vi "Set pin status.vi"(7 "Value":bool, 8 "error in (no error)":errorcluster, 9 "Pin":dbl, 10 "Port":dbl, 11 "Simulado in":refnum<class "Simulado.lvclass">) -> (0 "error out":errorcluster, 3 "Simulado out":refnum<class "Simulado.lvclass">)   [LabVIEW 2020, in "Simulado.lvclass"]
uses:
  Simulado.lvclass
  Simulado.lvclass/Simulado.ctl
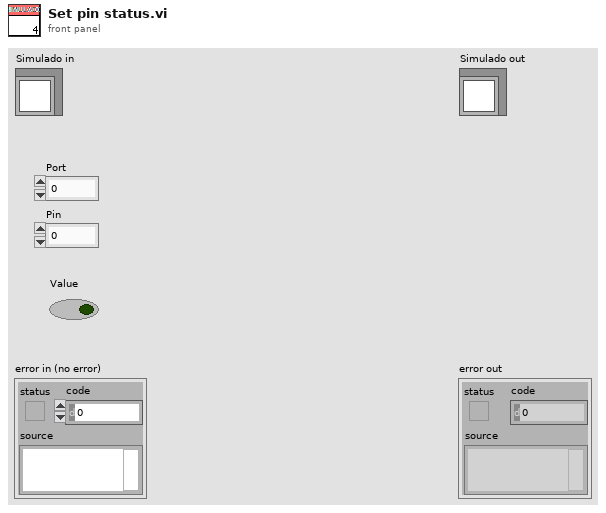
[diagram p1: front panel]
types:
  T1 = enum16{"reset parameters", "Get parameters", "Set parameter"}
  T2 = typedef "Serial Device.lvclass/serial device brand.ctl" = string
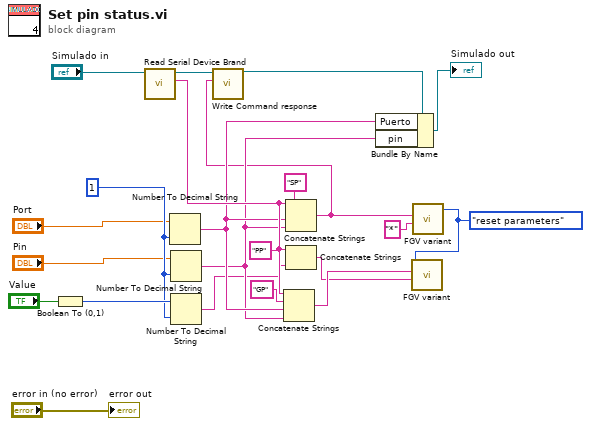
[diagram p0: block diagram]
diagram:
  w6 = T1."reset parameters" ("Functions")
  w15 = 1
  n1 = Boolean To (0,1)(Boolean="Value") -> (0, 1=w17:i16)
  n2 = call-dynamic "Read Serial Device Brand.vi"("Serial Device in"="Simulado in") -> ("Serial Device Brand"=w12:T2, "Serial Device out"=w21:refnum<class "Simulado.lvclass">)  [unwired: 8 in, 1 out]
  n3 = Number To Decimal String(number="Port", width (-)=w15) -> (decimal integer string=w8:string)
  n4 = Number To Decimal String(number="Pin", width (-)=w15) -> (decimal integer string=w7:string)
  n5 = Number To Decimal String(number=w17, width (-)=w15) -> (decimal integer string=w5:string)
  n6 = Concatenate Strings(w12, "GP" ("string"), w8, w7) -> (w3:string)
  n7 = Concatenate Strings(w12, "SP" ("string"), w8, w7) -> (w1:string)
  n8 = call-dynamic "Write Command response.vi"("Command response"=w1, "Simulado in"=w21) -> ("Simulado out"=w20:refnum<class "Simulado.lvclass">)  [unwired: 8 in, 1 out]
  n9 = Concatenate Strings(w12, "PP" ("string"), w5) -> (w2:string)
  n10 = Bundle By Name(cluster=w20, "Puerto"=w8, "pin"=w7) -> (→"Simulado out":refnum<class "Simulado.lvclass">)
  n11 = call "FGV variant.vi"("Response to save"=w2, "Command"=w3, "Functions"=w6) -> ()  [unwired: 7 in, 2 out]
  n12 = call "FGV variant.vi"("Response to save"="*", "Command"=w1, "Functions"=w6) -> ()  [unwired: 7 in, 2 out]
  "error out" <- "error in (no error)"
